vi "XBox Drive.vi"() -> (0 "XBox":T1)   [LabVIEW 2014]
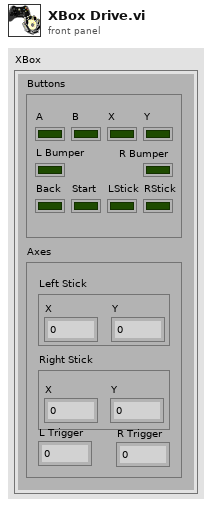
[diagram p1: front panel]
types:
  T1 = cluster{"Buttons":cluster{"A":bool, "B":bool, "X":bool, "Y":bool, "L Bumper":bool, "R Bumper":bool, "Back":bool, "Start":bool, "LStick":bool, "RStick":bool}, "Axes":cluster{"Left Stick":cluster{"X":dbl, "Y":dbl}, "Right Stick":cluster{"X":dbl, "Y":dbl}, "L Trigger":dbl, "R Trigger":dbl}}
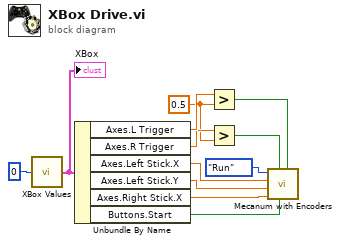
[diagram p0: block diagram]
diagram:
  w3 = 0.5 ("y")
  n1 = call "XBox Values.vi"("Index"=0) -> ("XBox"=w11:T1)
  "XBox" <- w11
  n2 = Unbundle By Name(w11) -> ("Axes.L Trigger"=w5:dbl, "Axes.R Trigger"=w4:dbl, "Axes.Left Stick.X"=w9:dbl, "Axes.Left Stick.Y"=w8:dbl, "Axes.Right Stick.X"=w7:dbl, "Buttons.Start"=w6:bool)
  n3 = Greater?(x=w5, y=w3) -> (0:w2:bool)
  n4 = Greater?(x=w4, y=w3) -> (0:w1:bool)
  n5 = call "Mecanum with Encoders.vi"("Slow?"=w2, "Reset"=w6, "Fast?"=w1, "Turn"=w7, "Forward/Backward"=w8, "Strafe"=w9, "Mode"=enum8{"Start", "Run", "Finish"}."Run") -> ()  [unwired: 3 in, 1 out]
